vi "LaunchTestPanel.vi"(7 "Wait Until Completion (T)?":bool=TRUE, 8 "Error In":errorcluster, 11 "Device name In":string) -> (0 "Error Out":errorcluster)   [LabVIEW 2011]
doc: "This VI will launch MAX Testpanel according to Device name."
panel:
  in  "ModuleType In":string
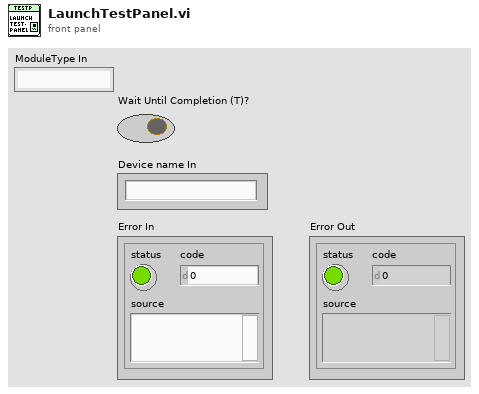
[diagram p1: front panel]
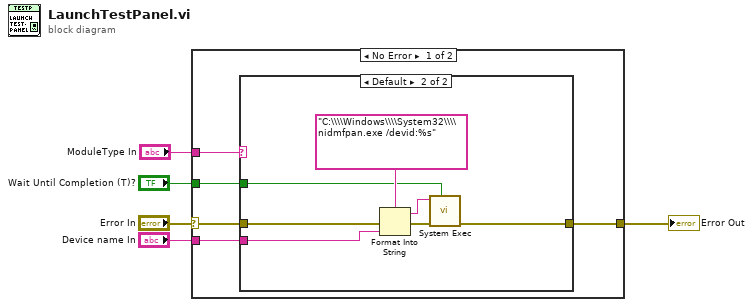
[diagram p0: block diagram]
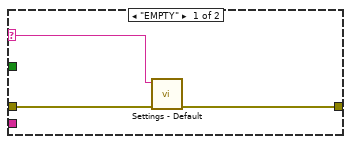
[diagram p2: hidden frame]
diagram:
  n1 = case shown="No Error" "Error In" {
    selector: "Error In" -> [w7 w21]
    tunnel: "Device name In" -> [w10 _]
    tunnel: [w9 w21] -> w4
    tunnel: "Wait Until Completion (T)?" -> [w8 _]
    tunnel: "ModuleType In" -> [w6 _]
    frame No Error {
      n2 = case shown="Default" w6 {
        selector: w6 -> [w11 _]
        tunnel: w10 -> [_ w19]
        tunnel: [w12 w17] -> w9
        tunnel: w8 -> [_ w15]
        tunnel: w7 -> [w13 w14]
        frame "EMPTY" {
          n3 = call "Settings - Default.vi"("Error In"=w13, "Module Name In"=w11) -> ("Error Out"=w12:errorcluster)  [unwired: 8 in, 1 out]
        }
        frame Default {
          n4 = Format Into String(format string="C:\\\\Windows\\\\System32\\\\nidmfpan.exe /devid:%s" ("command line"), error in=w14, w19) -> (resulting string=w20:string, error out=w18:errorcluster)  [unwired: 1 in]
          n5 = call <vilib>:"System Exec.vi"("wait until completion? (T)"=w15, "error in (no error)"=w18, "command line"=w20) -> ("error out"=w17:errorcluster)  [unwired: 5 in, 3 out]
        }
      }
    }
    frame Error {
    }
  }
  "Error Out" <- w4
